vi "MT EbN0 Calculation(MSK).vi"(0 "Recieved waveform":T3={"t0"=0.0, "dt"=1.0, "Y"=[]} {"Y" format="%.3f"; "dt" format="%^.2e"; "t0" format="%.4f"}, 1 "pulse shaping filter coefficients":dbl[](array[numeric]) format="%.2f", 5 "MSK system parameters":T1={"differential encoding enable"=enum."enable", "samples per symbol (16)"=16}, 7 "synchronization parameters":T2 {"sync sequence" format="%.2f"}, 9 "matched filter coefficients":dbl[](array[numeric]) format="%.2f", 11 "error in (no error)":errorcluster, 12 "reset? (T)":bool=TRUE) -> (4 "Eb/N0":dbl, 6 "Eb/N0(dB)":dbl, 15 "error out":errorcluster)   [LabVIEW 2020, in "niDMT.lvlib"]
uses:
  <vilib>/addons/Modulation/niDMT.lvlib
  <vilib>/addons/Modulation/Analog/controls/Complex Data Waveform.ctl
  <vilib>/addons/Modulation/niAMT.lvlib
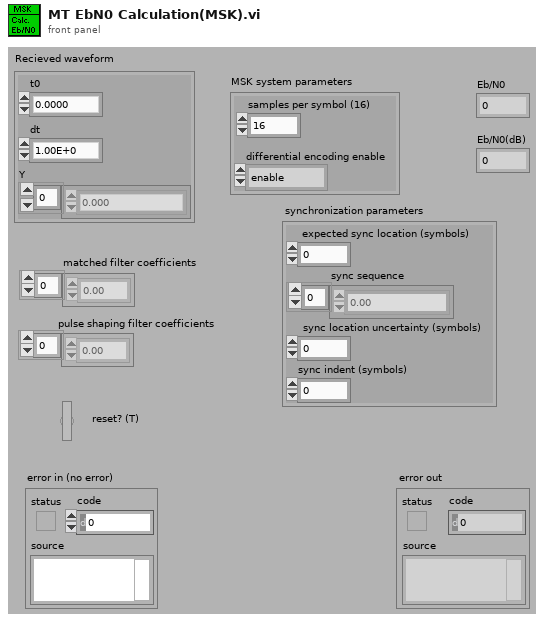
[diagram p1: front panel]
types:
  T1 = cluster{"differential encoding enable":enum16{"disable", "enable"}, "samples per symbol (16)":i32}
  T2 = cluster{"expected sync location (symbols)":i32, "sync sequence":cdb[], "sync location uncertainty (symbols)":i32, "sync indent (symbols)":i32}
  T3 = typedef "niAMT.lvlib/Complex Data Waveform.ctl" = cluster{"t0":dbl, "dt":dbl, "Y":cdb[]}
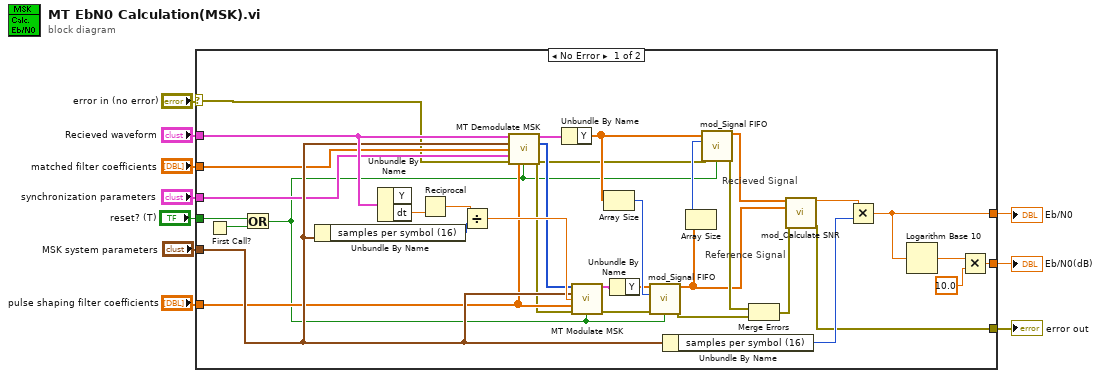
[diagram p0: block diagram]
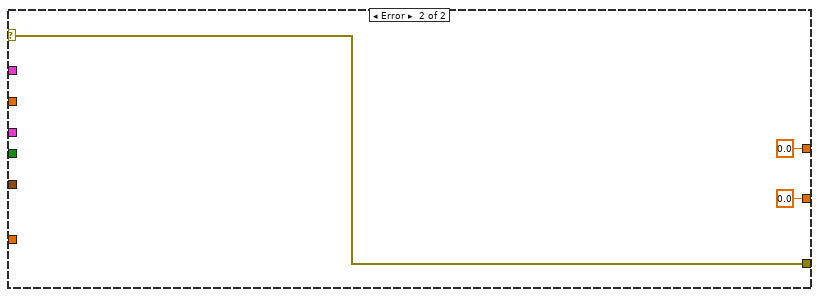
[diagram p2: hidden frame]
diagram:
  n1 = case shown="No Error" "error in (no error)" {
    selector: "error in (no error)" -> [w14 w45]
    tunnel: "Recieved waveform" -> [w39 _]
    tunnel: "MSK system parameters" -> [w38 _]
    tunnel: "synchronization parameters" -> [w37 _]
    tunnel: "matched filter coefficients" -> [w36 _]
    tunnel: "pulse shaping filter coefficients" -> [w35 _]
    tunnel: [w25 0.0] -> w5
    tunnel: [w24 0.0] -> w4
    tunnel: [w16 w45] -> w3
    tunnel: "reset? (T)" -> [w13 _]
    frame No Error {
      # "Recieved Signal"
      # "Reference Signal"
      n2 = First Call?() -> (First Call?: T/F=w12:bool)
      n3 = Or(x=w13, y=w12) -> (x .or. y?=w11:bool)
      n4 = Unbundle By Name(w38) -> ("samples per symbol (16)"=w42:i32)
      n5 = Unbundle By Name(w39) -> ("dt"=w44:dbl)  [unwired: 1 out]
      n6 = Reciprocal(x=w44) -> (1/x=w40:dbl)
      n7 = Divide(x=w40, y=w42) -> (x/y=w43:dbl)
      n8 = call <vilib>:"MT Demodulate MSK.vi"("input complex waveform"=w39, "MSK system parameters"=w38, "matched filter coefficients"=w36, "synchronization parameters"=w37, "error in (no error)"=w14, "pulse shaping filter coefficients"=w35, "reset? (T)"=w11) -> ("recovered complex waveform"=w33:T3, "output bit stream"=w34:i8[], "error out"=w23:errorcluster)  [unwired: 6 out]
      n9 = Unbundle By Name(w33) -> ("Y"=w31:cdb[])
      n10 = call <vilib>:"MT Modulate MSK.vi"("input bit stream"=w34, "MSK system parameters"=w38, "symbol rate (Hz)"=w43, "pulse shaping filter coefficients"=w35, "error in (no error)"=w23, "reset? (T)"=w11) -> ("output complex waveform"=w32:T3, "error out"=w22:errorcluster)  [unwired: 1 in, 7 out]
      n11 = Array Size(array=w31) -> (size(s)=w30:i32)
      n12 = Unbundle By Name(w32) -> ("Y"=w29:cdb[])
      n13 = call <vilib>:"mod_Signal FIFO.vi"("Signal In"=w29, "Output Length"=w30, "error in (no error)"=w22, "Reset? (T)"=w11) -> ("Signal Out"=w18:cdb[], "error out"=w20:errorcluster)  [unwired: 10 out]
      n14 = Unbundle By Name(w38) -> ("samples per symbol (16)"=w41:i32)
      n15 = Array Size(array=w18) -> (size(s)=w28:i32)
      n16 = call <vilib>:"mod_Signal FIFO.vi"("Signal In"=w31, "Output Length"=w28, "error in (no error)"=w23, "Reset? (T)"=w11) -> ("Signal Out"=w19:cdb[], "error out"=w21:errorcluster)  [unwired: 10 out]
      n17 = Merge Errors(w21, w20) -> (w17:errorcluster)
      n18 = call <vilib>:"mod_Calculate SNR.vi"("Recieved Waveform"=w19, "Reference Waveform"=w18, "error in (no error)"=w17) -> ("SNR"=w15:dbl, "error out"=w16:errorcluster)  [unwired: 11 out]
      n19 = Multiply(x=w15, y=w41) -> (x*y=w24:dbl)
      n20 = Logarithm Base 10(1:w24) -> (0:w27:dbl)
      n21 = Multiply(x=w27, y=10.0) -> (x*y=w25:dbl)
    }
    frame Error {
    }
  }
  "Eb/N0" <- w4
  "Eb/N0(dB)" <- w5
  "error out" <- w3
